vi "Hora_Limite.vi"(3 "Asc Reta RA rad":dbl=-0.383237875, 4 "Sideral Time rad":dbl=-0.383237875, 5 "Declinação rad":dbl=-0.383237875) -> (2 "TO Tempo de Observação Horas":dbl=-0.383237875)   [LabVIEW 2012]
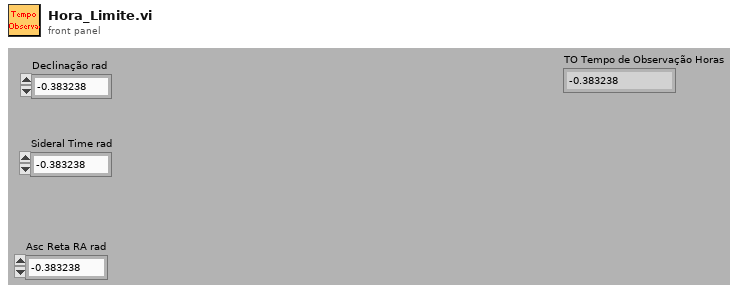
[diagram p1: front panel]
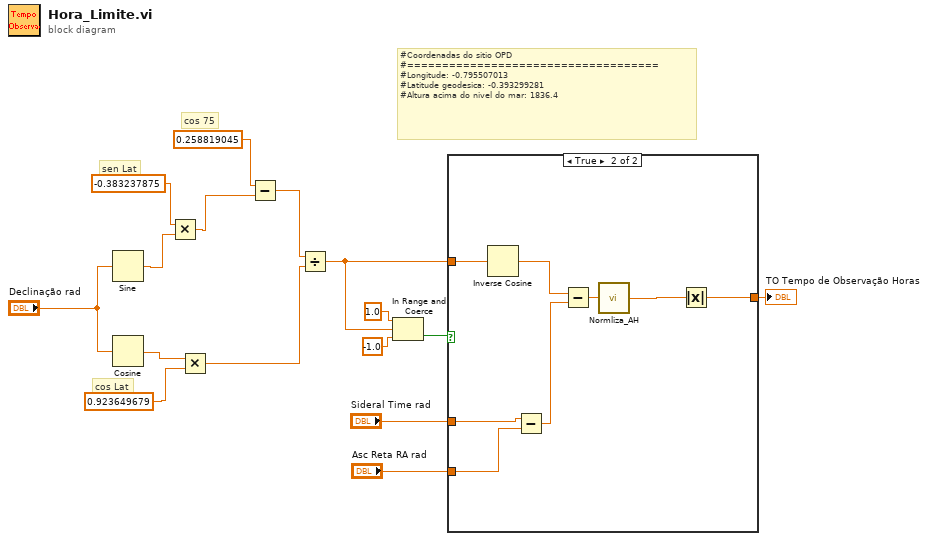
[diagram p0: block diagram]
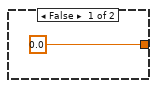
[diagram p2: hidden frame]
diagram:
  # "#Coordenadas do sitio OPD\n#====================================\n#Longitude: -0.795507013\n#Latitude geodesica: -0.393299281\n#Altura acima do nivel do mar: 1836.4"
  # "sen Lat"
  # "cos Lat"
  # "cos 75"
  n1 = Sine(x="Declinação rad") -> (sin(x)=w14:dbl)
  n2 = Cosine(x="Declinação rad") -> (cos(x)=w10:dbl)
  n3 = Multiply(x=-0.383237875, y=w14) -> (x*y=w12:dbl)
  n4 = Multiply(x=w10, y=0.923649679) -> (x*y=w8:dbl)
  n5 = Subtract(x=0.258819045, y=w12) -> (x-y=w11:dbl)
  n6 = Divide(x=w11, y=w8) -> (x/y=w2:dbl)
  n7 = In Range and Coerce(upper limit=1.0, x=w2, lower limit=-1.0) -> (In Range?=w1:bool)  [unwired: 1 out]
  n8 = case shown="True" w1 {
    tunnel: "Sideral Time rad" -> [_ w25]
    tunnel: "Asc Reta RA rad" -> [_ w24]
    tunnel: [0.0 ("t") w18] -> w5
    tunnel: w2 -> [_ w21]
    frame False {
    }
    frame True {
      n9 = Inverse Cosine(1:w21) -> (0:w22:dbl)
      n10 = Subtract(x=w25, y=w24) -> (x-y=w23:dbl)
      n11 = Subtract(x=w22, y=w23) -> (x-y=w20:dbl)
      n12 = call "Normliza_AH.vi"("PosAH"=w20) -> ("Numeric"=w19:dbl)
      n13 = Absolute Value(x=w19) -> (abs(x)=w18:dbl)
    }
  }
  "TO Tempo de Observação Horas" <- w5
